vi "Interface Write.vi"(8 "error in":errorcluster, 9 "timeout":i32=10000, 10 "data":u8[](array[numeric]), 11 "protocol layer in":refnum<class "Serial Interface.lvclass">) -> (0 "error out":errorcluster, 1 "timed out?":bool, 3 "protocol layer out":refnum<class "Serial Interface.lvclass">)   [LabVIEW 2021, in "Serial Interface.lvclass"]
doc: "This provides an interface for writing to a network bus."
uses:
  Serial Interface.lvclass
  Serial Interface.lvclass/Serial Interface.ctl
  Network Protocol/Serial Shared Components/Serial Shared Components.lvlib
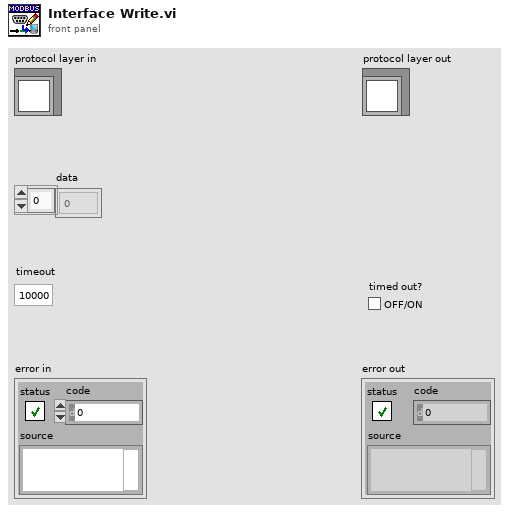
[diagram p1: front panel]
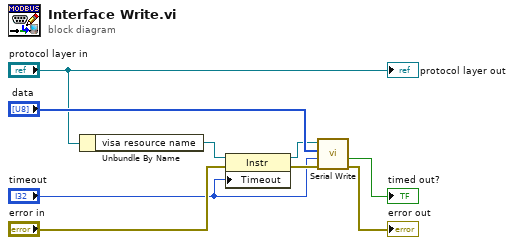
[diagram p0: block diagram]
diagram:
  n1 = Unbundle By Name("protocol layer in") -> ("visa resource name"=w3:refnum<visa-resource-name>)
  n2 = property class="Instr"(reference=w3, error in="error in", "Timeout"="timeout") -> (reference out=w2:refnum<visa-resource-name>, error out=w4:errorcluster)
  n3 = call "Serial Write.vi"("error in"=w4, "timeout (ms)"="timeout", "data"="data", "Visa Resource"=w2) -> ("error out"=→"error out":errorcluster, "timed out?"=→"timed out?":bool)  [unwired: 6 in]
  "protocol layer out" <- "protocol layer in"
